vi "Result File.vi"(10 "File Type":string, 11 "DesignRequest":T1) -> (2 "File string":string, 3 "File path":path)   [LabVIEW 2015]
uses:
  Design Request.ctl
  Variable cluster.ctl
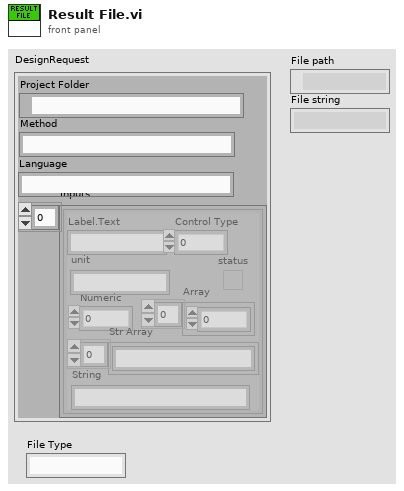
[diagram p1: front panel]
types:
  T1 = typedef "Design Request.ctl" = cluster{"Project Folder":path, "Method":string, "Inputs":T2, "Language":string}
  T2 = typedef "Variable cluster.ctl" = cluster{"Label.Text":string, "Control Type":u32, "Numeric":dbl, "Array":dbl[], "status":bool, "Str Array":string[], "String":string, "unit":string}[]
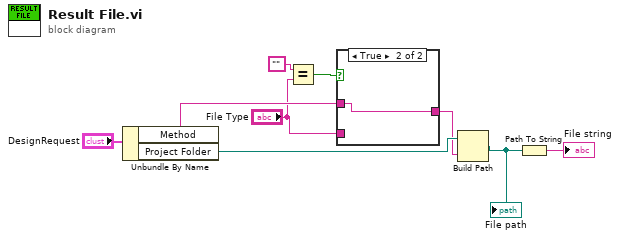
[diagram p0: block diagram]
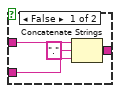
[diagram p2: hidden frame]
diagram:
  n1 = Unbundle By Name("DesignRequest") -> ("Method"=w5:string, "Project Folder"=w8:path)
  n2 = Equal?(x="", y="File Type") -> (x = y?=w2:bool)
  n3 = case shown="True" w2 {
    tunnel: "File Type" -> [w13 _]
    tunnel: [w12 w14] -> w6
    tunnel: w5 -> [w11 w14]
    frame False {
      n4 = Concatenate Strings(w11, "." ("string"), w13) -> (w12:string)
    }
    frame True {
    }
  }
  n5 = Build Path(base path=w8, name or relative path=w6) -> (appended path=w9:path)
  "File path" <- w9
  n6 = Path To String(path=w9) -> (string=→"File string":string)
